vi "Run VI.vi"(6 "Buildlog":path, 8 "error in (no error)":errorcluster, 11 "VI Path":path) -> (0 "error out":errorcluster)   [LabVIEW 2011]
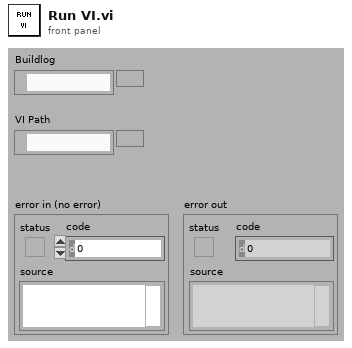
[diagram p1: front panel]
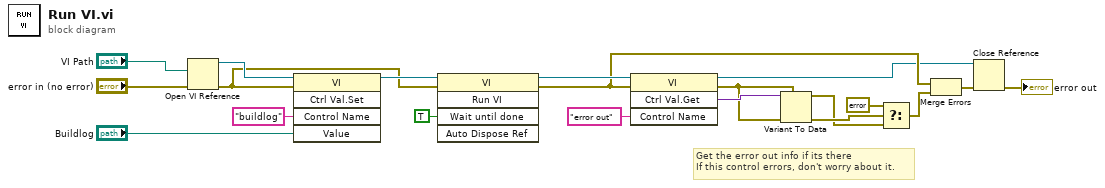
[diagram p0: block diagram]
diagram:
  # "Get the error out info if its there\nIf this control errors, don't worry about it."
  n1 = Open VI Reference(vi path="VI Path", error in (no error)="error in (no error)") -> (vi reference=w4:refnum<vi>, error out=w2:errorcluster)  [unwired: 4 in]
  n2 = invoke class="VI" method="Ctrl Val.Set"(reference=w4, error in=w2, "Control Name"="buildlog", "Value"="Buildlog") -> (reference out=w3:refnum<vi>)  [unwired: 1 in, 4 out]
  n3 = invoke class="VI" method="Run VI"(reference=w3, error in=w2, "Wait until done"=TRUE ("Wait Until Done")) -> (reference out=w17:refnum<vi>, error out=w10:errorcluster)  [unwired: 2 in, 3 out]
  n4 = invoke class="VI" method="Ctrl Val.Get"(reference=w17, error in=w10, "Control Name"="error out") -> (reference out=w6:refnum<vi>, error out=w14:errorcluster, "Get Control Value Variant"=w15:variant)  [unwired: 1 in, 1 out]
  n5 = Variant To Data(error in=w14, type=w14, Variant=w15) -> (data=w11:errorcluster, error out=w13:errorcluster)
  n6 = Select(t=errorcluster {"status"=FALSE, "code"=0, "source"=""}, s=w13, f=w11) -> (s? t:f=w9:errorcluster)
  n7 = Merge Errors(w10, w9) -> (w8:errorcluster)
  n8 = Close Reference(reference=w6, error in (no error)=w8) -> (error out=→"error out":errorcluster)
